vi "Get 2D CXT.vi"(7 "key description":string, 8 "sections":string[](array[string]), 9 "numeric":cxt[][](array[numeric]), 11 "info data":string) -> (0 "sections out":string[](array[string]), 1 "key found?":bool, 2 "value":cxt[][](array[numeric]) format="%.2f", 3 "info data out":string)   [LabVIEW 2020, in "infolib.lvlib"]
doc: "Reads matrix of CXT values. If section is entered it searches the key in the section(s).\nInput 'numeric' can be used to set default value.\nIf key is not found, the output value is equal to 'numeric' input.\nIf key is found, and element of matrix cannot be converted into data type, the default value of output matrix element is based on:\n- first element of 'numeric' input if available\n- otherwise NaN + NaN*i is used."
uses:
  infolib.lvlib
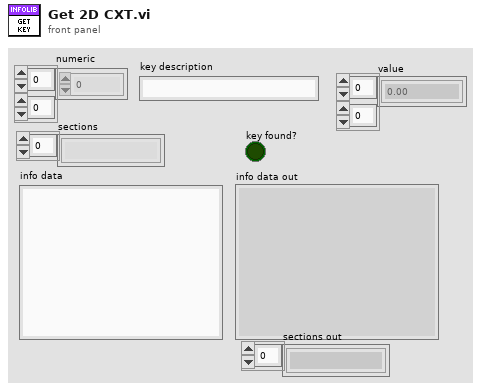
[diagram p1: front panel]
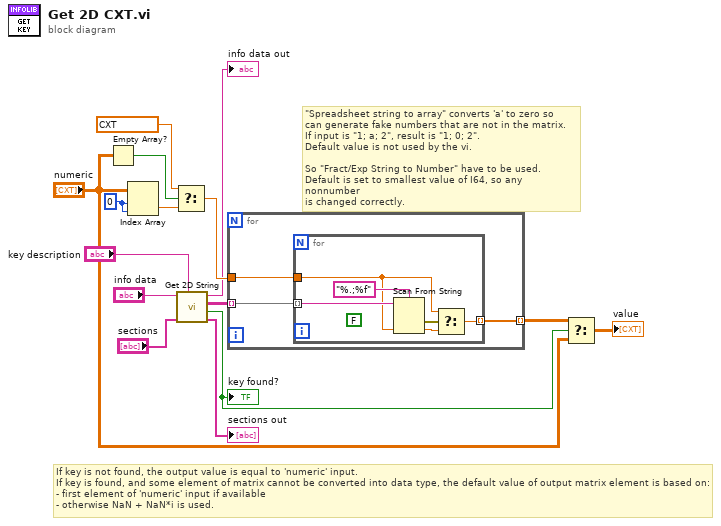
[diagram p0: block diagram]
diagram:
  w13 = 0 ("index (row)")
  # "If key is not found, the output value is equal to 'numeric' input.\nIf key is found, and some element of matrix cannot be converted into data type, the default value of output matrix element is based on:\n- first element of 'numeric' input if available\n- otherwise NaN + NaN*i is used."
  # "\"Spreadsheet string to array\" converts 'a' to zero so\ncan generate fake numbers that are not in the matrix.\nIf input is \"1; a; 2\", result is \"1; 0; 2\".\nDefault value is not used by the vi.\n\nSo \"Fract/Exp String to Number\" have to be used.\nDefault is set to smallest value of I64, so any nonnumber\nis changed correctly."
  n1 = Empty Array?(array="numeric") -> (empty?=w11:bool)
  n2 = Index Array(array="numeric", index (row)=w13, index (col)=w13) -> (element=w12:cxt)
  n3 = Select(t=cxt nan+nani ("x + iy"), s=w11, f=w12) -> (s? t:f=w8:cxt)
  n4 = call "Get 2D String.vi"("key description"="key description", "sections"="sections", "info data"="info data") -> ("sections out"=→"sections out":string[], "key found?"=w7:bool, "value"=w1:string[][], "info data out"=→"info data out":string)  [unwired: 5 in]
  "key found?" <- w7
  n5 = for {
    tunnel: w1 -> [w18] mode=indexing
    tunnel: [w17] -> w14 mode=indexing
    tunnel: w8 -> [w16]
    n6 = for {
      tunnel: w18 -> [w23] mode=indexing
      tunnel: [w21] -> w17 mode=indexing
      tunnel: w16 -> [w19]
      (unwired) FALSE ("use system decimal point (T)")
      n7 = Scan From String(format string="%.;%f", input string=w23, default 1=w19) -> (error out=w22:errorcluster, output 1=w20:cxt)  [unwired: 2 in, 2 out]
      n8 = Select(t=w19, s=w22, f=w20) -> (s? t:f=w21:cxt)
    }
  }
  n9 = Select(t=w14, s=w7, f="numeric") -> (s? t:f=→"value":cxt[][])
